vi "GD.vi"(2 "BMP File Path":path, 3 "XML indicator's config Path":path, 4 "XML File Path":path) -> (0 "vi refnum":refnum<vi>, 1 "toChanger":T1(array[cluster]))   [LabVIEW 2009]
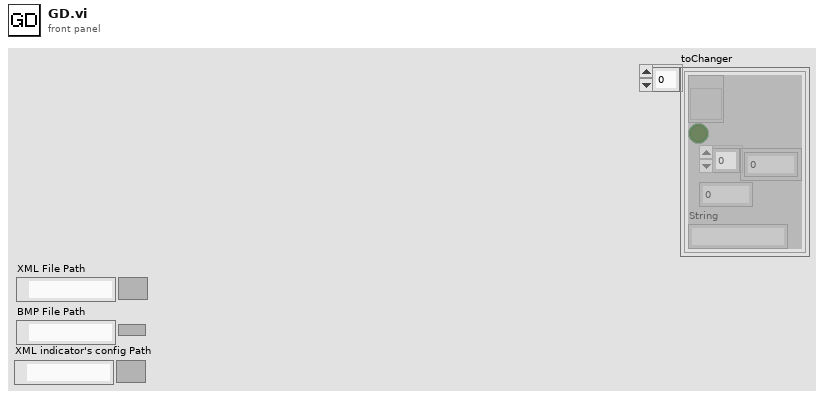
[diagram p1: front panel]
types:
  T1 = cluster{refnum<vi>, bool, i32[], i32, "String":string}[]
  T2 = cluster{"node text":string, cluster{"[0]":i32, "[1]":i32}, i32[], bool, bool, cluster{"[0]":u32, "[1]":u32}[], i32, "String":string, bool, i32, i32, i32, "node text":string, cluster{i32, i32}}[]
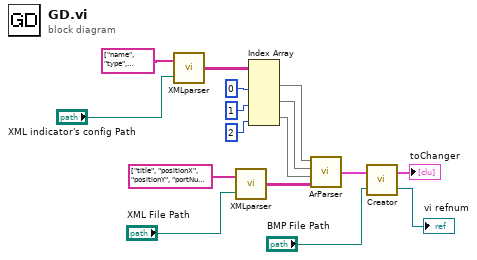
[diagram p0: block diagram]
diagram:
  n1 = call "XMLparser.vi"("XML File Path"="XML indicator's config Path", "Array"=string[] ["name", "type", "class"]) -> ("toArrayParser"=w10:string[][])
  n2 = call "XMLparser.vi"("XML File Path"="XML File Path", "Array"=string[] ["title", "positionX", "positionY", "portNum", "portType", "colorTrue", "colorFalse", "type", "bitNum", "minRange", "difRange", "heigth", "wigth"]) -> ("toArrayParser"=w3:string[][])
  n3 = Index Array(array=w10, index (col) #1=0 ("index (row)"), index (col) #2=1 ("index (row)"), index (col) #3=2 ("index (row)")) -> (element #1=w6:string[], element #2=w5:string[], element #3=w4:string[])  [unwired: 3 in]
  n4 = call "ArParser.vi"("from\nXMLparser"=w3, "IndicatorClasses"=w4, "IndicatorTypes"=w5, "IndicatorNames"=w6) -> ("toCreator"=w2:T2)
  n5 = call "Creator.vi"("BMP File Path"="BMP File Path", "toCreator"=w2) -> ("subvi"=→"vi refnum":refnum<vi>, "toChanger"=→"toChanger":T1)
